vi "Query IO.vi"(8 "error in":errorcluster, 11 "FPGA-DIO in":refnum<class "FPGA_DIO.lvclass">) -> (0 "error out":errorcluster, 1 "Port Array":u8[](array[numeric]), 2 "Boolean Array":bool[](array[boolean]), 3 "FPGA-DIO out":refnum<class "FPGA_DIO.lvclass">)   [LabVIEW 2019, in "FPGA_DIO.lvlib" / "FPGA_DIO.lvclass"]
doc: "This method must be overridden by the child class.\n\nThis should read the status at the output of the device and return a weform capture of the named signal states."
uses:
  Library/FPGA_DIO.lvclass
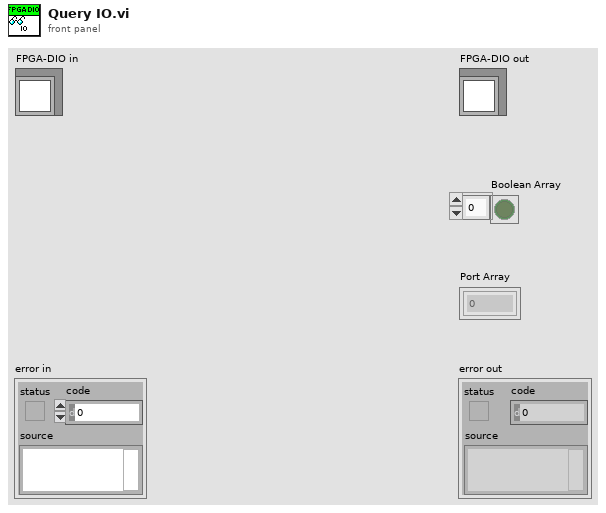
[diagram p1: front panel]
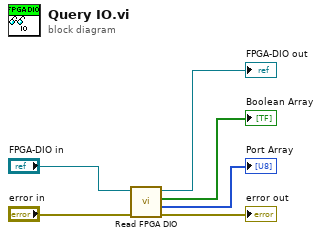
[diagram p0: block diagram]
diagram:
  n1 = call "Read FPGA DIO.vi"("error in"="error in", "FPGA-DIO in"="FPGA-DIO in") -> ("error out"=→"error out":errorcluster, "Port Array"=→"Port Array":u8[], "Boolean array"=→"Boolean Array":bool[], "FPGA-DIO out"=→"FPGA-DIO out":refnum<class "FPGA_DIO.lvclass">)  [unwired: 6 in]
